vi "Set Manual Mode.vi"(8 "error in (no error)":errorcluster, 9 "Power":dbl, 10 "Manual Mode":bool, 11 "Lakeshore 331 in":refnum<class "Lakeshore 331.lvclass">) -> (0 "error out":errorcluster, 3 "Lakeshore 331 out":refnum<class "Lakeshore 331.lvclass">)   [LabVIEW 2022 SP3, in "Lakeshore 331.lvclass"]
uses:
  Lakeshore 331.lvclass
  Lakeshore 331.lvclass/Lakeshore 331.ctl
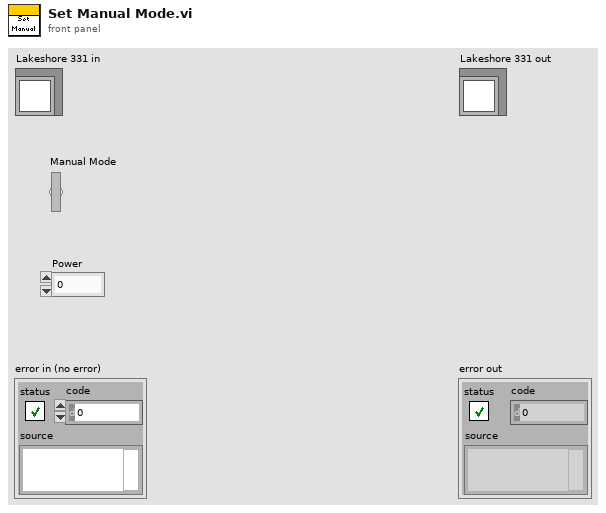
[diagram p1: front panel]
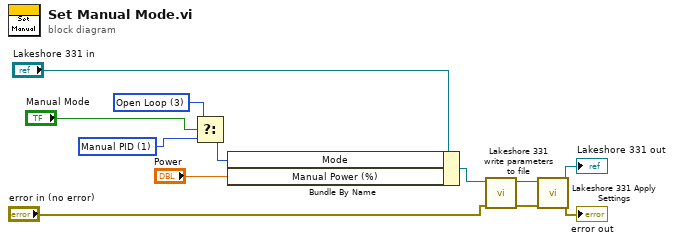
[diagram p0: block diagram]
diagram:
  w11 = u16 1 items=["Manual PID"=1, "Zone"=2, "Open Loop"=3, "AutoTune PID"=4, "AutoTune PI"=5, "AutoTune P"=6] ("Mode (1:Manual PID)")
  w12 = u16 3 items=["Manual PID"=1, "Zone"=2, "Open Loop"=3, "AutoTune PID"=4, "AutoTune PI"=5, "AutoTune P"=6] ("Mode (1:Manual PID)")
  n1 = Select(t=w12, s="Manual Mode", f=w11) -> (s? t:f=w10:u16)
  n2 = Bundle By Name(cluster="Lakeshore 331 in", "Mode"=w10, "Manual Power (%)"="Power") -> (w6:refnum<class "Lakeshore 331.lvclass">)
  n3 = call "Lakeshore 331 write parameters to file.vi"("error in (no error)"="error in (no error)", "Lakeshore 331 in"=w6) -> ("error out"=w3:errorcluster, "Lakeshore 331 out"=w5:refnum<class "Lakeshore 331.lvclass">)  [unwired: 8 in]
  n4 = call "Lakeshore 331 Apply Settings.vi"("error in (no error)"=w3, "Lakeshore 331 in"=w5) -> ("error out"=→"error out":errorcluster, "Lakeshore 331 out"=→"Lakeshore 331 out":refnum<class "Lakeshore 331.lvclass">)  [unwired: 8 in]
